vi "Example Command to gRPC.vi"(8 "error in (no error)":errorcluster, 10 "Command Data":i32, 11 "TemplatePlugin in":refnum<class "TemplatePlugin.lvclass">) -> (0 "error out":errorcluster, 3 "TemplatePlugin out":refnum<class "TemplatePlugin.lvclass">)   [LabVIEW 2021, in "TemplatePlugin.lvclass"]
uses:
  TemplatePlugin.lvclass
  TemplatePlugin.lvclass/TemplatePlugin.ctl
  8779bfbf-2797-4940-8d62-f4162e828731.vi
  cb651c69-5256-45bc-b9b0-1818fa9c55ac.vi
  Common/Typedef/OOB Comm/To gRPC Command.ctl
  Common/TemplateCommon.lvlib
  Common/Typedef/OOB Comm/To gRPC Command Data.ctl
  Common/Typedef/OOB Comm/To gRPC Command Payload.ctl
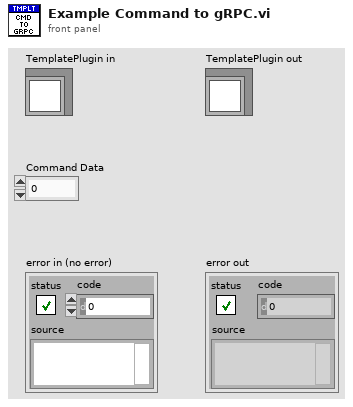
[diagram p1: front panel]
types:
  T1 = typedef "TemplateCommon.lvlib/To gRPC Command Payload.ctl" = cluster{"-> gRPC Command":T2, "-> gRPC Data":T3}
  T2 = typedef "TemplateCommon.lvlib/To gRPC Command.ctl" = enum16{"Read Data", "Read DVR Data"}
  T3 = typedef "TemplateCommon.lvlib/To gRPC Command Data.ctl" = cluster{"Cmd Data 1 -> gRPC":i32}
  T4 = typedef "TemplateCommon.lvlib/To gRPC DVR Data.ctl" = cluster{"Data 1 DVR -> gRPC ":i32}
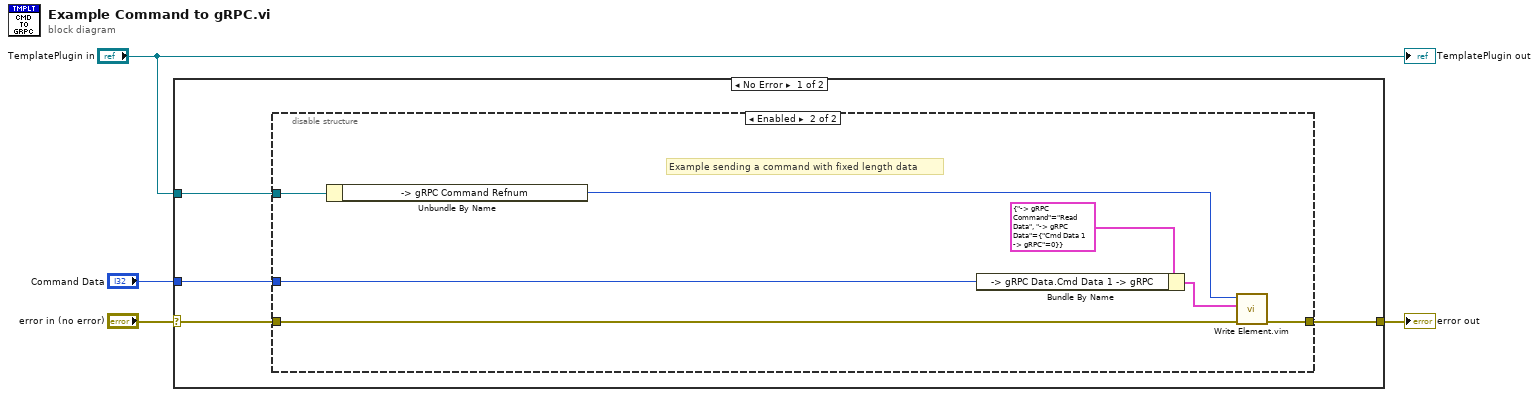
[diagram p0: block diagram]
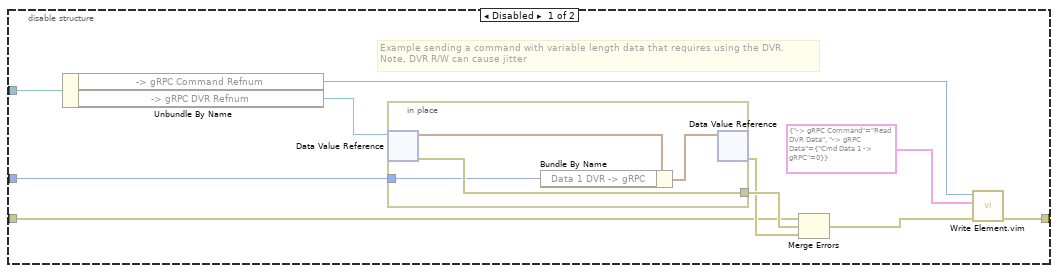
[diagram p2: hidden frame]
diagram:
  n1 = case shown="No Error" "error in (no error)" {
    selector: "error in (no error)" -> [w6 w30]
    tunnel: [w5 w30] -> w3
    tunnel: "TemplatePlugin in" -> [w8 _]
    tunnel: "Command Data" -> [w7 _]
    frame No Error {
      n2 = disable-structure shown="Enabled" {
        disable-tunnel: w8 -> [w13 w28]
        disable-tunnel: w7 -> [w12 w25]
        disable-tunnel: w6 -> [w11 w26]
        disable-tunnel: [w10 w27] -> w5
        frame Disabled {
          # "Example sending a command with variable length data that requires using the DVR.\nNote, DVR R/W can cause jitter"
          n3 = Unbundle By Name(w13) -> ("-> gRPC Command Refnum"=w15:u64, "-> gRPC DVR Refnum"=w18:refnum<data-value>)
          n4 = in-place {
            in-place-border: [w20] -> w16
            in-place-border: w12 -> [w19]
            n5 = in-place-dvr #1(w18) -> (w22:T4, w20:errorcluster)
            n6 = Bundle By Name(cluster=w22, "Data 1 DVR -> gRPC"=w19) -> (w21:T4)
            n7 = in-place-dvr #1(w21) -> (w14:errorcluster)  [unwired: 1 out]
          }
          n8 = Merge Errors(w11, w16, w14) -> (w17:errorcluster)
          n9 = call "Write Element.vim"("error in (no error)"=w17, "Data in"=T1 {"-> gRPC Command"=enum."Read DVR Data", "-> gRPC Data"={"Cmd Data 1 -> gRPC"=0}} ("-> gRPC Payload"), "CIPC Reference in"=w15) -> ("error out"=w10:errorcluster)  [unwired: 5 in, 3 out]
        }
        frame Enabled {
          # "Example sending a command with fixed length data"
          n10 = Unbundle By Name(w28) -> ("-> gRPC Command Refnum"=w29:u64)
          n11 = Bundle By Name(cluster=T1 {"-> gRPC Command"=enum."Read Data", "-> gRPC Data"={"Cmd Data 1 -> gRPC"=0}} ("-> gRPC Payload"), "-> gRPC Data.Cmd Data 1 -> gRPC"=w25) -> (w24:T1)
          n12 = call "Write Element.vim"("error in (no error)"=w26, "Data in"=w24, "CIPC Reference in"=w29) -> ("error out"=w27:errorcluster)  [unwired: 5 in, 3 out]
        }
      }
    }
    frame Error {
    }
  }
  "error out" <- w3
  "TemplatePlugin out" <- "TemplatePlugin in"
